vi "TalonSRXRPMtoNative100ms.vi"(4 "RPM":dbl) -> (1 "Velocity (Raw Sensor Units per 100 ms)":i32)   [LabVIEW 2019]
panel:
  in  "constant":dbl=0.146484375 format="%#_13g"
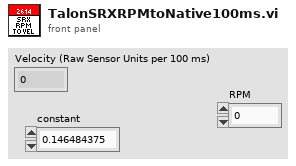
[diagram p1: front panel]
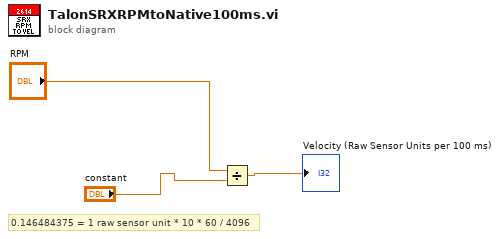
[diagram p0: block diagram]
diagram:
  # "0.146484375 = 1 raw sensor unit * 10 * 60 / 4096"
  n1 = Divide(x="RPM", y="constant") -> (x/y=→"Velocity (Raw Sensor Units per 100 ms)":dbl)
